vi "Convert Filter IDs Array to String.vi"(11 "Filter IDs":u32[](array[numeric])) -> (3 "Filter IDs":string caption="Filter IDs (format = x<ID>, comma seperated, ID x0 = Bus Error)")   [LabVIEW 2019, in "CAN Stream Support Workspace Shared.lvlib"]
uses:
  CAN Stream Support Workspace Shared.lvlib
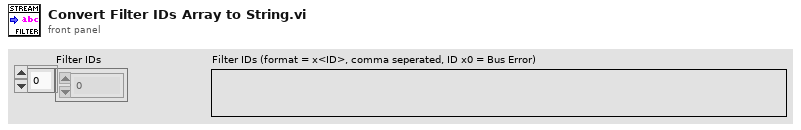
[diagram p1: front panel]
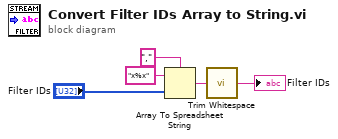
[diagram p0: block diagram]
diagram:
  n1 = Array To Spreadsheet String(delimiter (Tab)=",", array="Filter IDs", 3:"x%x" ("format string")) -> (spreadsheet string=w5:string)
  n2 = call <vilib>:"Trim Whitespace.vi"("string"=w5) -> ("trimmed string"=→"Filter IDs":string)  [unwired: 1 in]
